vi "CRYMultitone.vi"(0 "Stimulus Infor":T2={"Start Freq"=0.0, "Stop Freq"=0.0, "Step Number"=0, "Sweep Time"=0.0, "Level In"=0.0, "Cycles"=1.0, "Unit"=0, "Max"=0.0, "dB ref"=0.0} {"Cycles" max=3.0 step=1.0}, 2 "EQ Curve":T1={"Name"="", "Curve"=[], "X data"=1, "Y data"=1, "Z data"=1, "X axis"=0, "Y axis"=1, "Z axis"=1, "X unit"="Hz", "Y unit"="", "Z unit"="deg.", "X dB ref"=1.0, "Y dB ref"=1.0, "Z dB ref"=1.0, "single val"=FALSE, "protected"=FALSE, "display X"=TRUE, "display Y"=TRUE, "display Z"=TRUE, "Test Info"="", "Step No."=0, "Plot Settings"={"Color"=0, "Interpolation"=0, "Point Style"=0, "Line Style"=0, "Point Color"=0, "Line Width"=0, "Bar Plot Style"=0, "Fill To"=0}, "AutoProtect"=FALSE} {"Z data" items=["dB", "Lin"]; "X data" items=["dB", "Lin"]; "Y data" items=["dB", "Lin"]; "Z dB ref" format="%.1f"; "Z axis" items=["Log", "Lin"]; "X dB ref" format="%.1f"; "X axis" items=["Log", "Lin"]; "Y axis" items=["Log", "Lin"]; "Y dB ref" format="%.1f"; "Curve"."z" format="%.2f"; "Curve"."y" format="%.2f"; "Curve"."x" format="%.2f"}, 3 "Output Flag":cluster{bool, bool, "ApplyEQ":bool}, 5 "FAPS In":T3(array[cluster]), 7 "Fs":dbl, 9 "Resolution":u16, 11 "Freq Rounding":bool, 12 "Freq Rounding Value":dbl) -> (4 "tones":dbl[](array[numeric]) format="%.3f", 6 "FAPS":T3(array[cluster]), 15 "EQ Amplitude Rate":dbl)   [LabVIEW 2013]
uses:
  Typedef Control/CRYData Cluster.ctl
panel:
  out "max value 2":dbl
  out "max value":dbl
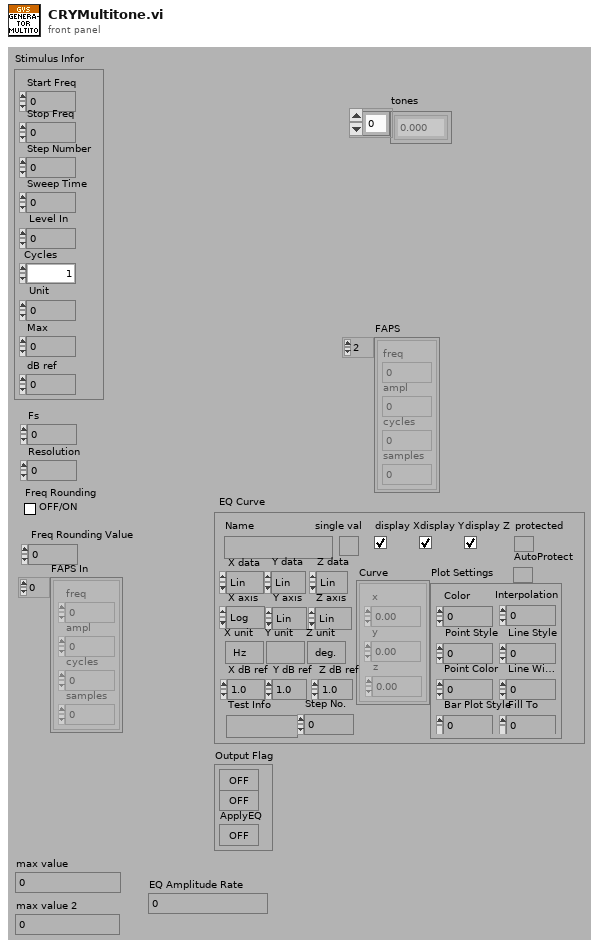
[diagram p1: front panel]
types:
  T1 = typedef "CRYData Cluster.ctl" = cluster{"Name":string, "Curve":cluster{"x":dbl, "y":dbl, "z":dbl}[], "X data":u16, "Y data":u16, "Z data":u16, "X axis":u16, "Y axis":u16, "Z axis":u16, "X unit":string, "Y unit":string, "Z unit":string, "X dB ref":dbl, "Y dB ref":dbl, "Z dB ref":dbl, "single val":bool, "protected":bool, "display X":bool, "display Y":bool, "display Z":bool, "Test Info":string, "Step No.":i32, "Plot Settings":cluster{"Color":u32, "Interpolation":u8, "Point Style":u8, "Line Style":u8, "Point Color":u32, "Line Width":u8, "Bar Plot Style":u8, "Fill To":i16}, "AutoProtect":bool}
  T2 = cluster{"Start Freq":dbl, "Stop Freq":dbl, "Step Number":u32, "Sweep Time":dbl, "Level In":dbl, "Cycles":dbl, "Unit":u16, "Max":dbl, "dB ref":dbl}
  T3 = cluster{"freq":dbl, "ampl":dbl, "cycles":dbl, "samples":i32}[]
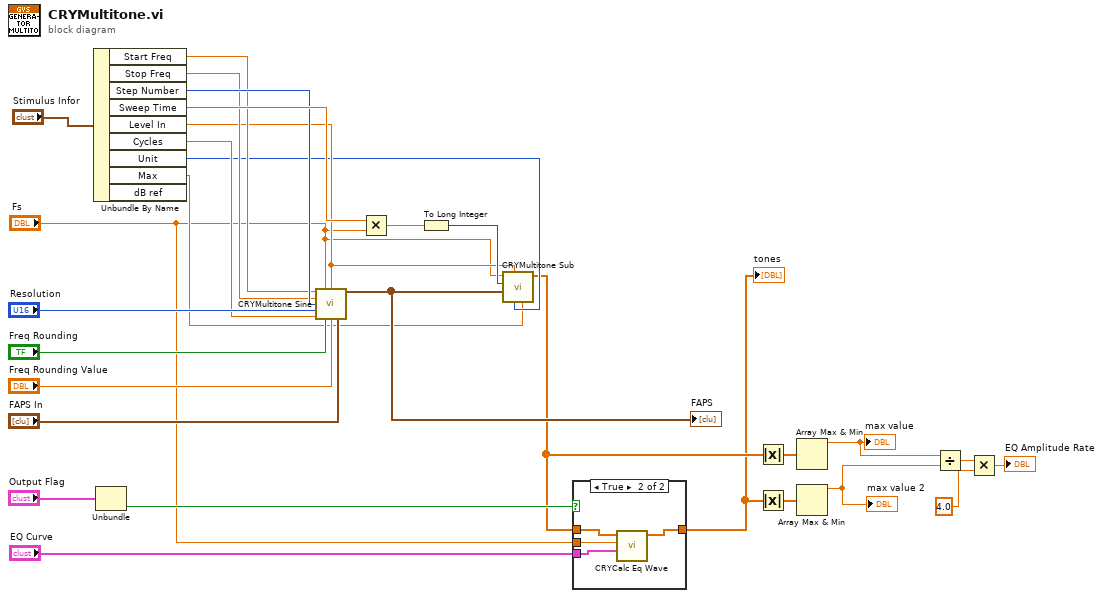
[diagram p0: block diagram]
diagram:
  n1 = Unbundle By Name("Stimulus Infor") -> ("Start Freq"=w19:dbl, "Stop Freq"=w18:dbl, "Step Number"=w20:u32, "Sweep Time"=w21:dbl, "Level In"=w16:dbl, "Cycles"=w17:dbl, "Unit"=w15:u16, "Max"=w14:dbl)  [unwired: 1 out]
  n2 = Unbundle("Output Flag") -> ("ApplyEQ"=w11:bool)  [unwired: 2 out]
  n3 = call "CRYMultitone Sine.vi"("Start Freq"=w19, "Fs"="Fs", "Level In"=w16, "Stop Freq"=w18, "Step Number"=w20, "Resolution"="Resolution", "Cycles"=w17, "Freq Rounding"="Freq Rounding", "Rounding value"="Freq Rounding Value", "FAPS In"="FAPS In") -> ("FAPS Out"=w26:T3)  [unwired: 1 in, 4 out]
  "FAPS" <- w26
  n4 = Multiply(x=w21, y="Fs") -> (x*y=w29:dbl)
  n5 = To Long Integer(number=w29) -> (32bit integer=w28:i32)
  n6 = call "CRYMultitone Sub.vi"("Max"=w14, "Level Type"=w15, "Level In"=w16, "FAPS"=w26, "samples"=w28, "Fs"="Fs") -> ("Multitone out"=w7:sgl[])  [unwired: 1 in, 4 out]
  n7 = case shown="True" w11 {
    tunnel: "EQ Curve" -> [_ w34]
    tunnel: "Fs" -> [_ w33]
    tunnel: w7 -> [w30 w32]
    tunnel: [w30 w31] -> w6
    frame False {
    }
    frame True {
      n8 = call "CRYCalc Eq Wave.vi"("EQ Curve"=w34, "Fs"=w33, "Wave In"=w32) -> ("Wave Out"=w31:dbl[])  [unwired: 7 in, 1 out]
    }
  }
  "tones" <- w6
  n9 = Absolute Value(x=w7) -> (abs(x)=w9:sgl[])
  n10 = Absolute Value(x=w6) -> (abs(x)=w8:dbl[])
  n11 = Array Max & Min(array=w9) -> (max value=w5:sgl)  [unwired: 3 out]
  "max value" <- w5
  n12 = Array Max & Min(array=w8) -> (max value=w4:dbl)  [unwired: 3 out]
  "max value 2" <- w4
  n13 = Divide(x=w5, y=w4) -> (x/y=w2:dbl)
  n14 = Multiply(x=w2, y=4.0) -> (x*y=→"EQ Amplitude Rate":dbl)
